vi "Export_map2Text v10.2.vi"(1 "MapData (2D)":dbl[][](array[numeric]), 2 "XY Full Interpolated":cluster{dbl, dbl}[](array[cluster]), 3 "ExportPath":path) -> ()   [LabVIEW 2010]
uses:
  <vilib>/Analysis/polynomials.llb/Unique Numbers and Multiplicity (DBL).vi
  <vilib>/Utility/file.llb/Write To Spreadsheet File (DBL).vi
  <vilib>/Analysis/NI_AALPro.lvlib
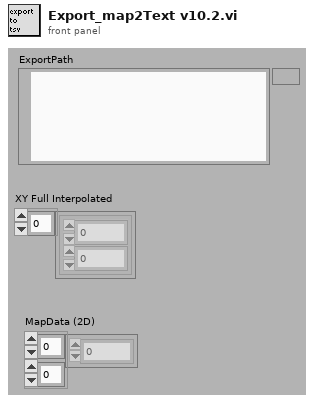
[diagram p1: front panel]
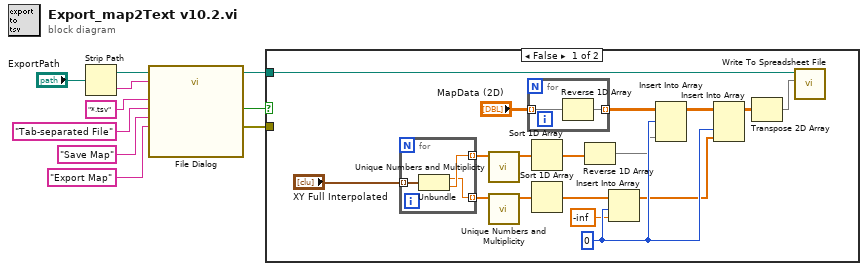
[diagram p0: block diagram]
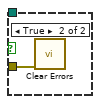
[diagram p2: hidden frame]
diagram:
  n1 = Strip Path(path="ExportPath") -> (stripped path=w6:path, name=w5:string)
  n2 = call "File Dialog"("start path"=w6, "prompt"="Export Map" ("button label"), "button label"="Save Map" ("prompt"), "default name"=w5, "pattern (all files)"="*.tsv", "pattern label"="Tab-separated File") -> ("selected path"=w10:path, "cancelled"=w9:bool, "error out"=w8:errorcluster)  [unwired: 6 in, 1 out]
  n3 = case shown="False" w9 {
    tunnel: w10 -> [w27 _]
    tunnel: w8 -> [_ w33]
    frame False {
      w25 = 0 ("Deaktivierter Index (Spalte)")
      n4 = for {
        tunnel: "XY Full Interpolated" -> [w32] mode=indexing
        tunnel: [w30] -> w12 mode=indexing
        tunnel: [w31] -> w11 mode=indexing
        n5 = Unbundle(w32) -> (w30:dbl, w31:dbl)
      }
      n6 = call-poly <vilib>:"Unique Numbers and Multiplicity.vi"("Numbers"=w11) -> ("Unique Numbers"=w21:dbl[])  [unwired: 8 in, 2 out]
      n7 = call-poly <vilib>:"Unique Numbers and Multiplicity.vi"("Numbers"=w12) -> ("Unique Numbers"=w22:dbl[])  [unwired: 8 in, 2 out]
      n8 = for {
        tunnel: "MapData (2D)" -> [w29] mode=indexing
        tunnel: [w28] -> w13 mode=indexing
        n9 = Reverse 1D Array(array=w29) -> (reversed array=w28:dbl[])
      }
      n10 = Sort 1D Array(array=w21) -> (sorted array=w16:dbl[])
      n11 = Sort 1D Array(array=w22) -> (sorted array=w19:dbl[])
      n12 = Reverse 1D Array(array=w16) -> (reversed array=w15:dbl[])
      n13 = Insert Into Array(array=w19, index=w25, new element=-inf ("Neues Element/Teil-Array")) -> (w23:dbl[])
      n14 = Insert Into Array(array=w13, index (row)=w25, new element=w15) -> (w26:dbl[][])  [unwired: 1 in]
      n15 = Insert Into Array(array=w26, index (col)=w25, new element=w23) -> (w18:dbl[][])  [unwired: 1 in]
      n16 = Transpose 2D Array(2D array=w18) -> (transposed array=w17:dbl[][])
      n17 = call-poly <vilib>:"Write To Spreadsheet File.vi"("2D data"=w17, "file path (dialog if empty)"=w27) -> ()  [unwired: 6 in, 1 out]
    }
    frame True {
      n18 = call <vilib>:"Clear Errors.vi"("error in (no error)"=w33) -> ()  [unwired: 6 in, 1 out]
    }
  }
